vi "DLSsetup.vi"(8 "error in (no error)":errorcluster, 10 "Delay Time":dbl[unit] format="%.3f", 11 "SEQ in":refnum<class "Sequence.lvclass">) -> (0 "error out":errorcluster, 3 "SEQ w/DT":T1)   [LabVIEW 2012, in "StimulCtrls.lvlib"]
uses:
  StimulCtrls.lvlib
  UserControl/ElectdPanel.ctl
  UserControl/ElectdTerminal.ctl
  Sequence.lvclass
panel:
  in  "Stop Button":bool
  out "Tag":string
  out "SEQ Panel":T4 {"Electrode 16"."Magnitude" format="%4.2f"; "Electrode 15"."Magnitude" format="%4.2f"; "Electrode 14"."Magnitude" format="%4.2f"; "Electrode 13"."Magnitude" format="%4.2f"; "Electrode 12"."Magnitude" format="%4.2f"; "Electrode 11"."Magnitude" format="%4.2f"; "Electrode 10"."Magnitude" format="%4.2f"; "Electrode 9"."Magnitude" format="%4.2f"; "Electrode 8"."Magnitude" format="%4.2f"; "Electrode 7"."Magnitude" format="%4.2f"; "Electrode 6"."Magnitude" format="%4.2f"; "Electrode 5"."Magnitude" format="%4.2f"; "Electrode 4"."Magnitude" format="%4.2f"; "Electrode 3"."Magnitude" format="%4.2f"; "Electrode 2"."Magnitude" format="%4.2f"; "Electrode"."Magnitude" format="%4.2f"}
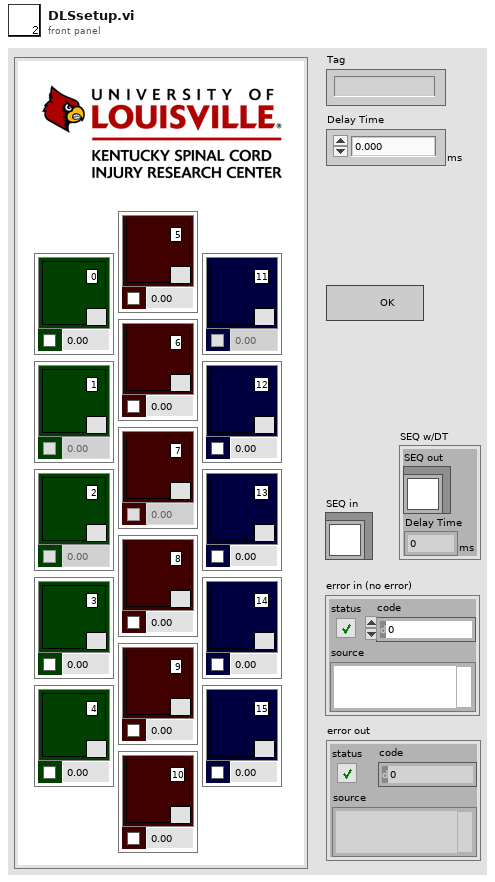
[diagram p1: front panel]
types:
  T1 = cluster{"SEQ out":refnum<class "Sequence.lvclass">, "Delay Time":dbl[unit]}
  T2 = typedef "StimulCtrls.lvlib/ElectdPanel.ctl" = cluster{"Group #":string, "T #":T3, "Magnitude":sgl, "check":bool}
  T3 = typedef "StimulCtrls.lvlib/ElectdTerminal.ctl" = u8
  T4 = cluster{"Electrode":T2, "Electrode 2":T2, "Electrode 3":T2, "Electrode 4":T2, "Electrode 5":T2, "Electrode 6":T2, "Electrode 7":T2, "Electrode 8":T2, "Electrode 9":T2, "Electrode 10":T2, "Electrode 11":T2, "Electrode 12":T2, "Electrode 13":T2, "Electrode 14":T2, "Electrode 15":T2, "Electrode 16":T2}
  T5 = cluster{"Sequence out":refnum<class "Sequence.lvclass">, "Delay Time":dbl[unit]}
  T6 = cluster{"SEQ in":refnum<class "Sequence.lvclass">, dbl[unit]}
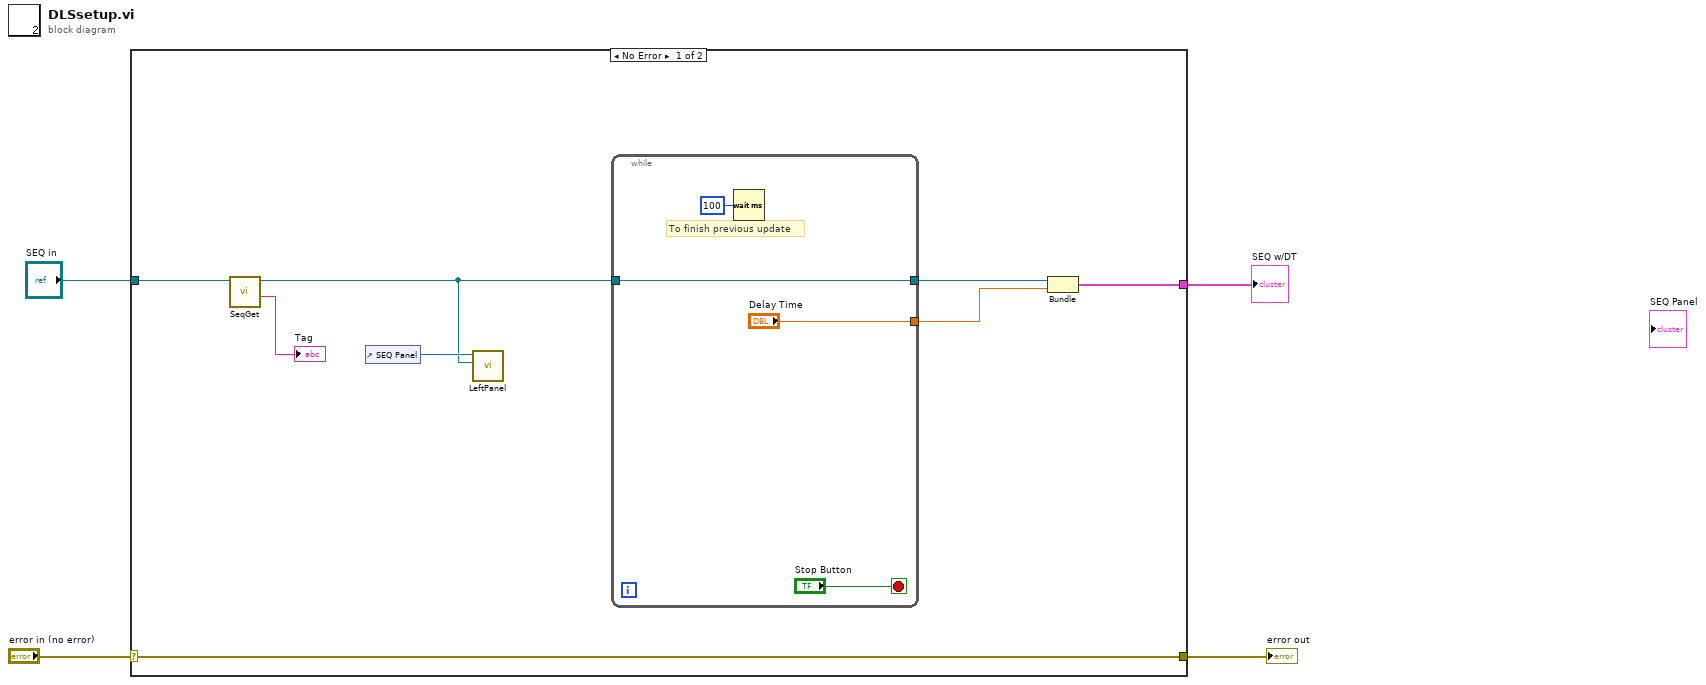
[diagram p0: block diagram]
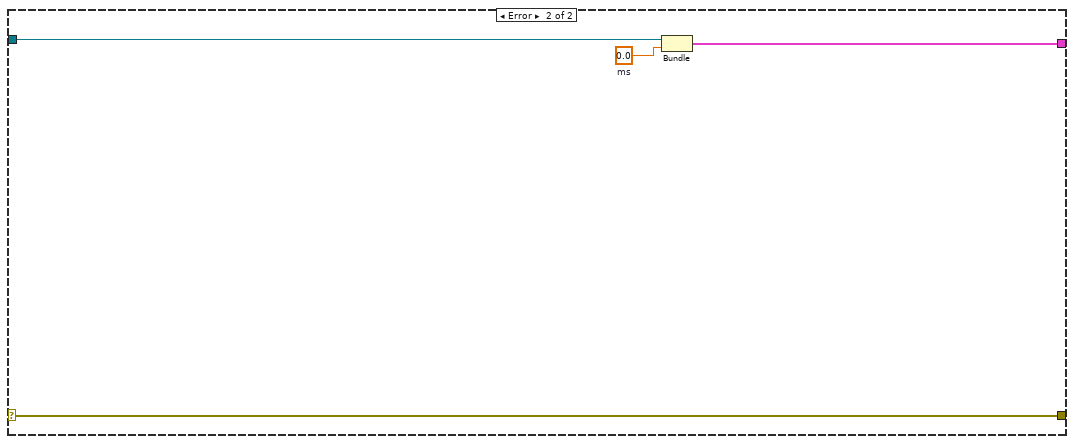
[diagram p2: hidden frame]
diagram:
  n1 = case shown="No Error" "error in (no error)" {
    selector: "error in (no error)" -> [w12 w20]
    tunnel: [w12 w20] -> w3
    tunnel: [w7 w17] -> w2
    tunnel: "SEQ in" -> [w9 w19]
    frame No Error {
      n2 = call-dynamic "SeqGet.vi"("Sequence in"=w9) -> ("Tag"=→"Tag":string, "Sequence out"=w8:refnum<class "Sequence.lvclass">)  [unwired: 7 in, 2 out]
      n3 = control-ref of="SEQ Panel"() -> (w10:refnum<vi>)
      n4 = call "LeftPanel.vi"("Seqn in"=w8, "Panel Refnum"=w10) -> ()  [unwired: 9 in]
      n5 = while {
        tunnel: [w15] -> w6
        tunnel: w8 -> [w15]
        tunnel: ["Delay Time"] -> w5
        stop <- "Stop Button" stop-if-true
        # "To finish previous update"
        n6 = Wait (ms)(milliseconds to wait=u32 100) -> ()  [unwired: 1 out]
      }
      n7 = Bundle("Sequence out"=w6, "Delay Time"=w5) -> (w7:T5)  [unwired: 1 in]
    }
    frame Error {
      w18 = dbl[unit] 0.0  # ms
      n8 = Bundle("SEQ in"=w19, w18) -> (w17:T6)  [unwired: 1 in]
    }
  }
  "error out" <- w3
  "SEQ w/DT" <- w2
